vi "Runtime.Transfer.Config to Runtime.vi"(8 "error in (no error)":errorcluster, 9 "Access":T1, 11 "Device Ref in":T2=18446744073709551615 format="%.0x") -> (0 "error out":errorcluster, 3 "Device Ref out":T2=18446744073709551615 format="%.0x")   [LabVIEW 2016, in "Data Sharing Framework Runtime API.lvlib"]
uses:
  Data Sharing Framework Runtime API.lvlib
  Classes/Runtime/Channel/Runtime.Channel.lvclass
  <vilib>/NI VeriStand/Custom Device API/Custom Device API.lvlib
  Classes/Configuration.Channel/Configuration.Channel.lvclass
  <vilib>/NI Veristand/VeriStand Data/VeriStand Data.lvlib
  <vilib>/NI Veristand/Custom Device API/Custom Device Item Ref.ctl
  <vilib>/NI Veristand/Custom Device API/Data Access Type.ctl
  Classes/Configuration.Transfer/Configuration.Transfer.lvclass
  Classes/Runtime/Transfer/Runtime.Transfer.lvclass
panel:
  in  "Transfer Runtime":refnum<class "Runtime.Transfer.lvclass">
  in  "Transfer Configuration":refnum<class "Configuration.Transfer.lvclass">
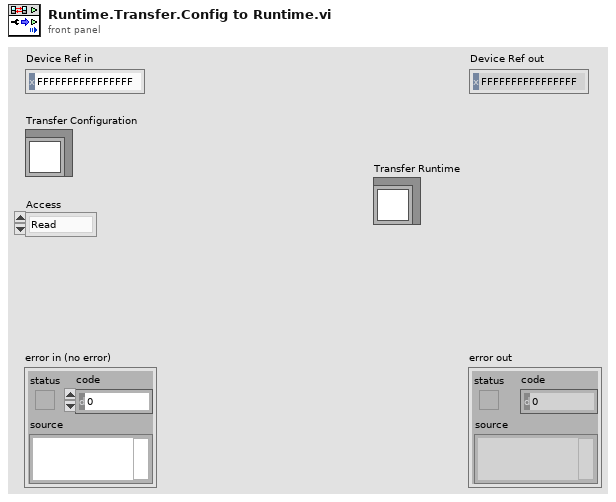
[diagram p1: front panel]
types:
  T1 = typedef "Custom Device API.lvlib/Data Access Type.ctl" = enum16{"Read", "Write"}
  T2 = typedef "Custom Device API.lvlib/Custom Device Item Ref.ctl" = u64
  T3 = typedef "VeriStand Data.lvlib/Typedefs.Data Types.ctl" = enum16{"Boolean", "Single", "Double", "I8", "I16", "I32", "I64", "U8", "U16", "U32", "U64"}
  T4 = typedef "Custom Device API.lvlib/Data Reference.ctl" = i32
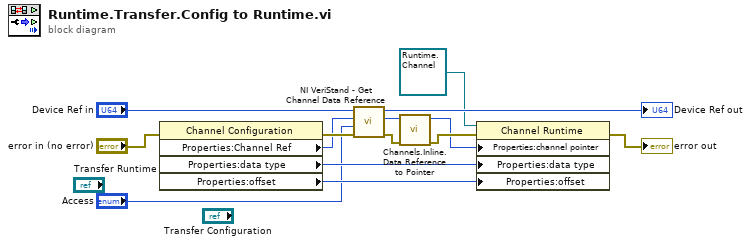
[diagram p0: block diagram]
diagram:
  n1 = property class="Channel Configuration"(error in="error in (no error)") -> (reference=w16:refnum<class "Configuration.Channel.lvclass">, error out=w15:errorcluster, "Properties:Channel Ref"=w14:T2, "Properties:data type"=w13:T3, "Properties:offset"=w12:u64)  [unwired: 1 out]
  n2 = call <vilib>:"NI VeriStand - Get Channel Data Reference.vi"("error in (no error)"=w15, "Access"="Access", "Channel Ref in"=w14, "Device Ref in"="Device Ref in") -> ("error out"=w5:errorcluster, "Channel Data Reference"=w4:T4, "Device Ref out"=→"Device Ref out":T2)  [unwired: 5 in]
  n3 = call <vilib>:"Channels.Inline.Data Reference to Pointer.vi"("error in (no error)"=w5, "Data Reference in"=w4) -> ("error out"=w3:errorcluster, "Channel Pointer"=w2:u64)  [unwired: 8 in]
  n4 = property class="Channel Runtime"(reference=refnum<class "Runtime.Channel.lvclass"> refnum ("Channel Runtime"), error in=w3, "Properties:channel pointer"=w2, "Properties:data type"=w13, "Properties:offset"=w12) -> (reference out=w11:refnum<class "Runtime.Channel.lvclass">, error out=→"error out":errorcluster)
